vi "Test Spreadsheet String To Array.vi"(8 "error in (no error)":errorcluster) -> (0 "error out":errorcluster, 3 "Pass?":bool)   [LabVIEW 2020]
uses:
  G-Unicode/Unicode/Controls/String Encoding.ctl
  G-Unicode/Types/UTF-8 String/UTF-8 String.lvclass
  G-Unicode/Types/UTF-8 String/UTF-8 String.lvclass/UTF-8 String.ctl
  cf201102-b386-4106-b0a3-b8bc94e6a325.vi
  eb18ccdd-5ad3-4b0e-afdf-25bd5b000ab7.vi
  bee85e8b-63c5-43ce-881d-e4e1380263d7.vi
  4f09a9e4-b4f8-42f0-b4ae-0eea3f0ba849.vi
  0eb54c82-1323-4bed-85ac-3c12f1ca81eb.vi
  4af515d9-751f-4e33-a134-290fcdfcef32.vi
  4ceb4ac6-5f19-4790-bb02-bb32d441528f.vi
  2bc9fe8b-6368-403f-a424-8bd266d475bb.vi
  ad1cb8aa-aa11-4123-a9f7-e3f12093d3f0.vi
  29dfd71c-33c6-4992-af8b-de78e3ac8f96.vi
  d42ab165-0845-4272-a91a-d7364413acc5.vi
  ac4c9d38-978d-4f5f-bde7-6196e55a1839.vi
  5e87d20b-6b60-47b6-90d0-1ac0ea1c11ff.vi
  1be032f7-2608-481d-a623-c0828a24587f.vi
  9f520168-cbc4-4090-a9f5-4e2f9dbbbb8b.vi
  c16da871-6a6c-4ecf-a232-eda9a31815a2.vi
  ddc13801-d6f6-4314-812d-5b78cce9f754.vi
  8662db80-a6bf-419e-a5ab-b32bcbb679d5.vi
  f65f8089-79d8-41df-af02-5220a5419b68.vi
  91528c36-808d-479b-a42b-6e92cf357bd2.vi
  73ebf715-1fe5-4766-95cc-638d64213c87.vi
  e78a3d6a-c4b5-4d57-bbf5-e1752e7799af.vi
  bd25557d-86f5-46fb-92bd-cfaa82f7c03f.vi
  G-Unicode/Unicode/Encode String.vi
  cf201102-b386-4106-b0a3-b8bc94e6a325.vi/46bf550a-28c6-4dfd-813a-9b0ad34779ef.vi
  G-Unicode/Private/Conversion/String as Encoded String.vi
  G-Unicode/Private/Conversion/Polymorphic VIs/String as Encoded String (UTF-8 String).vi
  G-Unicode/Types/UTF-8 String/Write Encoded UTF-8 String.vi
  eb18ccdd-5ad3-4b0e-afdf-25bd5b000ab7.vi/46bf550a-28c6-4dfd-813a-9b0ad34779ef.vi
  G-Unicode/Types/UTF-8 String/Read Encoded UTF-8 String.vi
  bee85e8b-63c5-43ce-881d-e4e1380263d7.vi/3a31b270-3bb6-4c58-a256-c5fcc2c98f09.vi
  bee85e8b-63c5-43ce-881d-e4e1380263d7.vi/0ec5df2d-ef9b-4f84-a6a8-ffcedd45c4dc.vi
  4f09a9e4-b4f8-42f0-b4ae-0eea3f0ba849.vi/46bf550a-28c6-4dfd-813a-9b0ad34779ef.vi
  0eb54c82-1323-4bed-85ac-3c12f1ca81eb.vi/46bf550a-28c6-4dfd-813a-9b0ad34779ef.vi
  4af515d9-751f-4e33-a134-290fcdfcef32.vi/3a31b270-3bb6-4c58-a256-c5fcc2c98f09.vi
  4af515d9-751f-4e33-a134-290fcdfcef32.vi/0ec5df2d-ef9b-4f84-a6a8-ffcedd45c4dc.vi
  4ceb4ac6-5f19-4790-bb02-bb32d441528f.vi/46bf550a-28c6-4dfd-813a-9b0ad34779ef.vi
  2bc9fe8b-6368-403f-a424-8bd266d475bb.vi/3a31b270-3bb6-4c58-a256-c5fcc2c98f09.vi
  2bc9fe8b-6368-403f-a424-8bd266d475bb.vi/0ec5df2d-ef9b-4f84-a6a8-ffcedd45c4dc.vi
  ad1cb8aa-aa11-4123-a9f7-e3f12093d3f0.vi/46bf550a-28c6-4dfd-813a-9b0ad34779ef.vi
  29dfd71c-33c6-4992-af8b-de78e3ac8f96.vi/46bf550a-28c6-4dfd-813a-9b0ad34779ef.vi
  d42ab165-0845-4272-a91a-d7364413acc5.vi/3a31b270-3bb6-4c58-a256-c5fcc2c98f09.vi
  d42ab165-0845-4272-a91a-d7364413acc5.vi/0ec5df2d-ef9b-4f84-a6a8-ffcedd45c4dc.vi
  ac4c9d38-978d-4f5f-bde7-6196e55a1839.vi/46bf550a-28c6-4dfd-813a-9b0ad34779ef.vi
  5e87d20b-6b60-47b6-90d0-1ac0ea1c11ff.vi/3a31b270-3bb6-4c58-a256-c5fcc2c98f09.vi
  5e87d20b-6b60-47b6-90d0-1ac0ea1c11ff.vi/0ec5df2d-ef9b-4f84-a6a8-ffcedd45c4dc.vi
  1be032f7-2608-481d-a623-c0828a24587f.vi/46bf550a-28c6-4dfd-813a-9b0ad34779ef.vi
  9f520168-cbc4-4090-a9f5-4e2f9dbbbb8b.vi/46bf550a-28c6-4dfd-813a-9b0ad34779ef.vi
  c16da871-6a6c-4ecf-a232-eda9a31815a2.vi/3a31b270-3bb6-4c58-a256-c5fcc2c98f09.vi
  c16da871-6a6c-4ecf-a232-eda9a31815a2.vi/0ec5df2d-ef9b-4f84-a6a8-ffcedd45c4dc.vi
  ddc13801-d6f6-4314-812d-5b78cce9f754.vi/46bf550a-28c6-4dfd-813a-9b0ad34779ef.vi
  8662db80-a6bf-419e-a5ab-b32bcbb679d5.vi/3a31b270-3bb6-4c58-a256-c5fcc2c98f09.vi
  8662db80-a6bf-419e-a5ab-b32bcbb679d5.vi/0ec5df2d-ef9b-4f84-a6a8-ffcedd45c4dc.vi
  f65f8089-79d8-41df-af02-5220a5419b68.vi/46bf550a-28c6-4dfd-813a-9b0ad34779ef.vi
  91528c36-808d-479b-a42b-6e92cf357bd2.vi/46bf550a-28c6-4dfd-813a-9b0ad34779ef.vi
  73ebf715-1fe5-4766-95cc-638d64213c87.vi/3a31b270-3bb6-4c58-a256-c5fcc2c98f09.vi
  73ebf715-1fe5-4766-95cc-638d64213c87.vi/0ec5df2d-ef9b-4f84-a6a8-ffcedd45c4dc.vi
  e78a3d6a-c4b5-4d57-bbf5-e1752e7799af.vi/46bf550a-28c6-4dfd-813a-9b0ad34779ef.vi
  bd25557d-86f5-46fb-92bd-cfaa82f7c03f.vi/3a31b270-3bb6-4c58-a256-c5fcc2c98f09.vi
  bd25557d-86f5-46fb-92bd-cfaa82f7c03f.vi/0ec5df2d-ef9b-4f84-a6a8-ffcedd45c4dc.vi
  G-Unicode/Private/Conversion/Text to UTF-8.vi
  G-Unicode/Private/Conversion/Polymorphic VIs/Text to UTF-8 (LabVIEW String).vi
  G-Unicode/Private/Conversion/Encoded UTF-8 String to Encoded UTF-16LE String.vi
  G-Unicode/Unicode/SubVIs/UTF-16 Byte Swap.vi
  G-Unicode/Private/Conversion/UTF-8 to Text.vi
  G-Unicode/Private/Conversion/Polymorphic VIs/UTF-8 to Text (LabVIEW String).vi
  G-Unicode/Private/Conversion/Encoded UTF-16LE String to Encoded UTF-8 String.vi
  G-Unicode/Unicode/Prepend BOM.vi
  G-Unicode/Private/Conversion/Polymorphic VIs/String as Encoded String (LabVIEW String).vi
  G-Unicode/Private/Conversion/Text as Encoded String.vi
  G-Unicode/Private/Conversion/Polymorphic VIs/Text as Encoded String (UTF-8 String).vi
  G-Unicode/Unicode/SubVIs/Byte Order Marks.vi
  G-Unicode/Unicode/Detect BOM.vi
  G-Unicode/Unicode/Detect String Encoding.vi
  G-Unicode/G-Unicode.lvlib
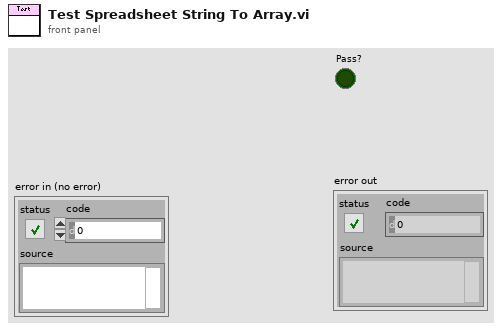
[diagram p1: front panel]
types:
  T1 = typedef "G-Unicode.lvlib/String Encoding.ctl" = enum16{"ANSI", "UTF-8", "UTF-16LE", "UTF-16BE", "Unknown"}
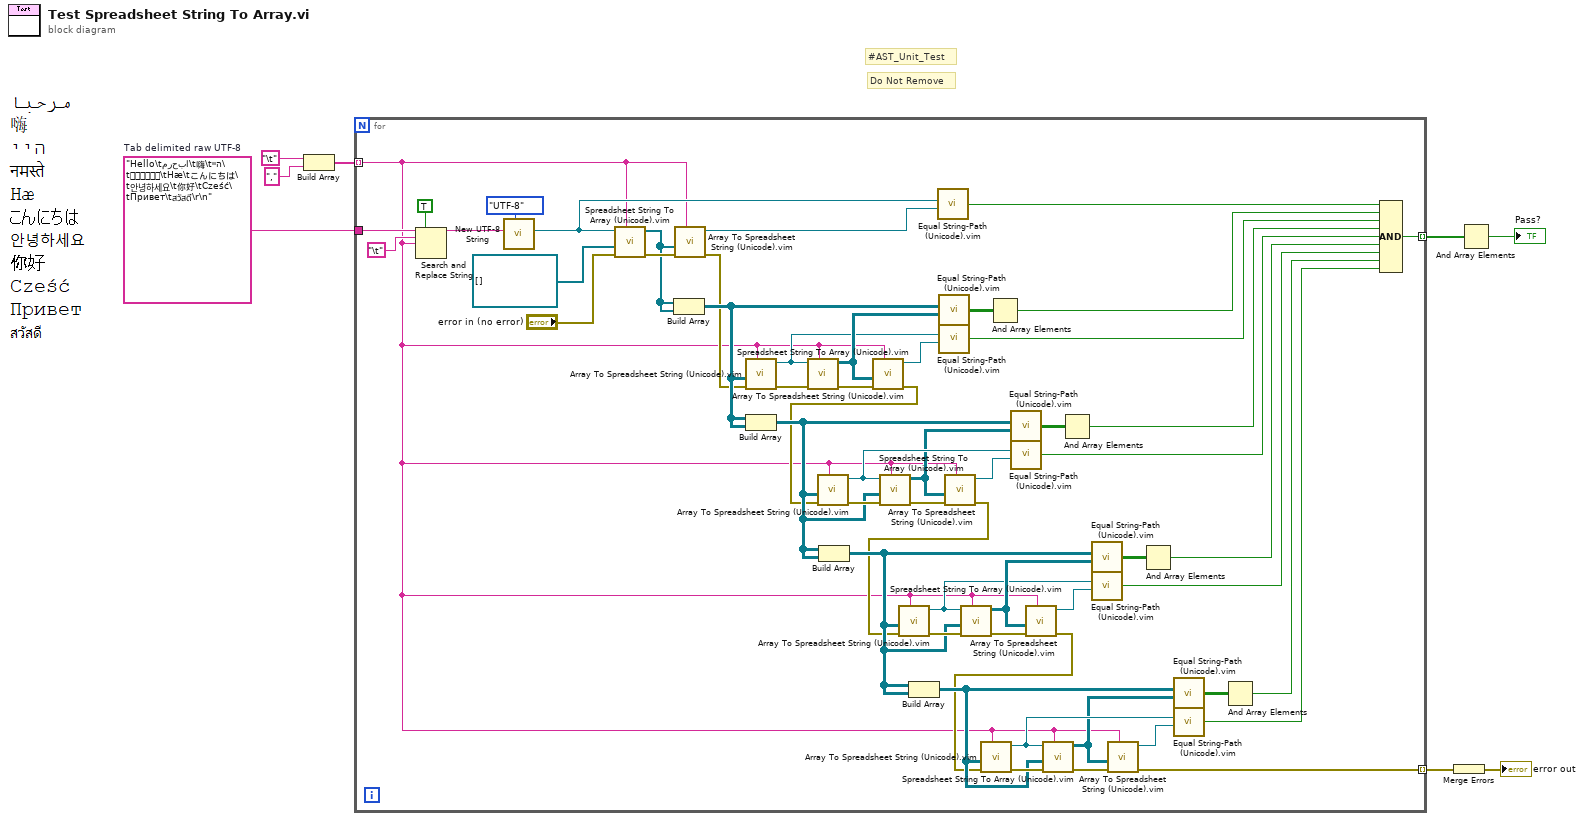
[diagram p0: block diagram]
diagram:
  w1 = "Hello\tمرحبا\t嗨\tהיי\tनमस्ते\tHæ\tこんにちは\t안녕하세요\t你好\tCześć\tПривет\tสวัสดี\r\n"  # Tab delimited raw UTF-8
  # "Do Not Remove"
  # "#AST_Unit_Test"
  n1 = Build Array("\t", "," ("element")) -> (w2:string[])
  n2 = for {
    tunnel: [w63] -> w8 mode=indexing
    tunnel: [w15] -> w7 mode=indexing
    tunnel: w1 -> [w13]
    tunnel: w2 -> [w9] mode=indexing
    n3 = Search and Replace String(replace all?=TRUE ("replace all? (F)"), input string=w13, search string="\t", replace string=w9) -> (result string=w12:string)  [unwired: 4 in, 3 out]
    n4 = call "New UTF-8 String.vi"("Input Encoding (ANSI)"=String_Encoding."UTF-8", "String"=w12) -> ("UTF-8 String"=w50:refnum<class "UTF-8 String.lvclass">)  [unwired: 8 in, 1 out]
    n5 = call "Spreadsheet String To Array (Unicode).vim"("Delimiter (tab)"=w9, "error in"="error in (no error)", "Array Type (2D UTF-8 String)"=refnum<class "UTF-8 String.lvclass">[] [], "Spreadsheet String"=w50) -> ("error out"=w59:errorcluster, "Array"=w41:refnum<class "UTF-8 String.lvclass">[])  [unwired: 6 in]
    n6 = Build Array(w41, w41) -> (w39:refnum<class "UTF-8 String.lvclass">[][])
    n7 = call "Array To Spreadsheet String (Unicode).vim"("Delimiter (tab)"=w9, "error in"=w59, "Array"=w41) -> ("error out"=w19:errorcluster, "Spreadsheet String"=w49:refnum<class "UTF-8 String.lvclass">)  [unwired: 7 in]
    n8 = call "Array To Spreadsheet String (Unicode).vim"("Delimiter (tab)"=w9, "error in"=w19, "Array"=w39) -> ("error out"=w60:errorcluster, "Spreadsheet String"=w55:refnum<class "UTF-8 String.lvclass">)  [unwired: 7 in]
    n9 = Build Array(w39, w39) -> (w32:refnum<class "UTF-8 String.lvclass">[][][])
    n10 = call "Spreadsheet String To Array (Unicode).vim"("Delimiter (tab)"=w9, "error in"=w60, "Spreadsheet String"=w55) -> ("error out"=w57:errorcluster, "Array"=w56:refnum<class "UTF-8 String.lvclass">[][])  [unwired: 7 in]
    n11 = Build Array(w32, w32) -> (w22:refnum<class "UTF-8 String.lvclass">[][][][])
    n12 = call "Array To Spreadsheet String (Unicode).vim"("Delimiter (tab)"=w9, "error in"=w57, "Array"=w56) -> ("error out"=w18:errorcluster, "Spreadsheet String"=w54:refnum<class "UTF-8 String.lvclass">)  [unwired: 7 in]
    n13 = call "Array To Spreadsheet String (Unicode).vim"("Delimiter (tab)"=w9, "error in"=w18, "Array"=w32) -> ("error out"=w44:errorcluster, "Spreadsheet String"=w46:refnum<class "UTF-8 String.lvclass">)  [unwired: 7 in]
    n14 = call "Spreadsheet String To Array (Unicode).vim"("Delimiter (tab)"=w9, "error in"=w44, "Array Type (2D UTF-8 String)"=w32, "Spreadsheet String"=w46) -> ("error out"=w45:errorcluster, "Array"=w40:refnum<class "UTF-8 String.lvclass">[][][])  [unwired: 6 in]
    n15 = Build Array(w22, w22) -> (w23:refnum<class "UTF-8 String.lvclass">[][][][][])
    n16 = call "Equal String-Path (Unicode).vim"("y"=w49, "x"=w50) -> ("Equal?"=w58:bool)  [unwired: 7 in, 1 out]
    n17 = call "Equal String-Path (Unicode).vim"("y"=w56, "x"=w39) -> ("Equal?"=w53:bool[][])  [unwired: 7 in, 1 out]
    n18 = call "Equal String-Path (Unicode).vim"("y"=w54, "x"=w55) -> ("Equal?"=w51:bool)  [unwired: 7 in, 1 out]
    n19 = call "Array To Spreadsheet String (Unicode).vim"("Delimiter (tab)"=w9, "error in"=w45, "Array"=w40) -> ("error out"=w17:errorcluster, "Spreadsheet String"=w47:refnum<class "UTF-8 String.lvclass">)  [unwired: 7 in]
    n20 = call "Array To Spreadsheet String (Unicode).vim"("Delimiter (tab)"=w9, "error in"=w17, "Array"=w22) -> ("error out"=w37:errorcluster, "Spreadsheet String"=w35:refnum<class "UTF-8 String.lvclass">)  [unwired: 7 in]
    n21 = call "Spreadsheet String To Array (Unicode).vim"("Delimiter (tab)"=w9, "error in"=w37, "Array Type (2D UTF-8 String)"=w22, "Spreadsheet String"=w35) -> ("error out"=w36:errorcluster, "Array"=w38:refnum<class "UTF-8 String.lvclass">[][][][])  [unwired: 6 in]
    n22 = And Array Elements(Boolean array=w53) -> (logical AND=w52:bool)
    n23 = call "Equal String-Path (Unicode).vim"("y"=w40, "x"=w32) -> ("Equal?"=w48:bool[][][])  [unwired: 7 in, 1 out]
    n24 = call "Equal String-Path (Unicode).vim"("y"=w47, "x"=w46) -> ("Equal?"=w42:bool)  [unwired: 7 in, 1 out]
    n25 = call "Array To Spreadsheet String (Unicode).vim"("Delimiter (tab)"=w9, "error in"=w36, "Array"=w38) -> ("error out"=w16:errorcluster, "Spreadsheet String"=w34:refnum<class "UTF-8 String.lvclass">)  [unwired: 7 in]
    n26 = call "Array To Spreadsheet String (Unicode).vim"("Delimiter (tab)"=w9, "error in"=w16, "Array"=w23) -> ("error out"=w25:errorcluster, "Spreadsheet String"=w27:refnum<class "UTF-8 String.lvclass">)  [unwired: 7 in]
    n27 = call "Spreadsheet String To Array (Unicode).vim"("Delimiter (tab)"=w9, "error in"=w25, "Array Type (2D UTF-8 String)"=w23, "Spreadsheet String"=w27) -> ("error out"=w26:errorcluster, "Array"=w24:refnum<class "UTF-8 String.lvclass">[][][][][])  [unwired: 6 in]
    n28 = And Array Elements(Boolean array=w48) -> (logical AND=w43:bool)
    n29 = call "Equal String-Path (Unicode).vim"("y"=w38, "x"=w22) -> ("Equal?"=w33:bool[][][][])  [unwired: 7 in, 1 out]
    n30 = call "Equal String-Path (Unicode).vim"("y"=w34, "x"=w35) -> ("Equal?"=w30:bool)  [unwired: 7 in, 1 out]
    n31 = call "Array To Spreadsheet String (Unicode).vim"("Delimiter (tab)"=w9, "error in"=w26, "Array"=w24) -> ("error out"=w15:errorcluster, "Spreadsheet String"=w28:refnum<class "UTF-8 String.lvclass">)  [unwired: 7 in]
    n32 = And Array Elements(Boolean array=w33) -> (logical AND=w31:bool)
    n33 = call "Equal String-Path (Unicode).vim"("y"=w24, "x"=w23) -> ("Equal?"=w29:bool[][][][][])  [unwired: 7 in, 1 out]
    n34 = call "Equal String-Path (Unicode).vim"("y"=w28, "x"=w27) -> ("Equal?"=w20:bool)  [unwired: 7 in, 1 out]
    n35 = And Array Elements(Boolean array=w29) -> (logical AND=w21:bool)
    n36 = Compound Arithmetic op=AND(w58, w52, w51, w43, w42, w31, w30, w21, w20) -> (w63:bool)
  }
  n37 = Merge Errors(w7) -> (→"error out":errorcluster)
  n38 = And Array Elements(Boolean array=w8) -> (logical AND=→"Pass?":bool)
